vi "IMAQdx LL-Snap.vi"(7 "ImgName":string="untitled", 8 "ErrIn":errorcluster) -> (0 "ErrOut":errorcluster, 3 "ImgOut":T1)   [LabVIEW 2013]
doc: "Use this template to build a VI to use as a subVI."
uses:
  <vilib>/vision/Image Controls.llb/IMAQ Image.ctl
  <vilib>/vision/driver/IMAQdx.llb/IMAQdx Acquisition Mode.ctl
  <vilib>/vision/driver/IMAQdx.llb/IMAQdx Buffer Number Mode.ctl
  <vilib>/vision/driver/NI_Vision_Acquisition_Software.lvlib
panel:
  in  "Camera":refnum<k21> caption="IMAQdx Session"
  # "Input Parameters"
  # "Output Parameters"
  # "VI Description:\nThis VI is created to snap a image from imaging device."
  # ":: MVI Framework V1.0 ::\nAuthor:Gaoke Yang\nEmail: gaoke.yang@yahoo.com\nWeb: www.mvicontrol.com\nCopyright (C) 2013, MVI Technologies All Rights Reserved"
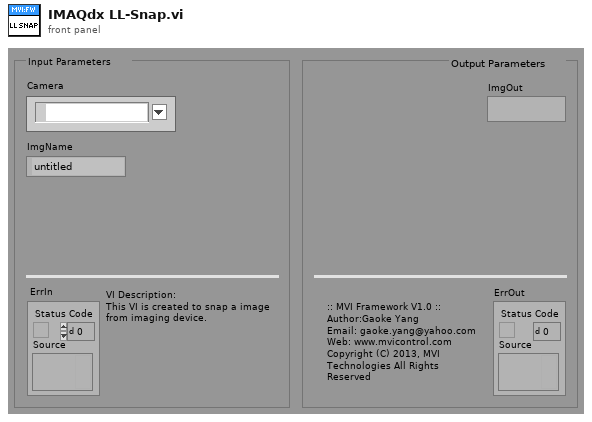
[diagram p1: front panel]
types:
  T1 = typedef "IMAQ Image.ctl" = refnum<image>
  T2 = typedef "NI_Vision_Acquisition_Software.lvlib/IMAQdx Buffer Number Mode.ctl" = enum32{"Next", "Last", "Buffer Number"}
  T3 = typedef "NI_Vision_Acquisition_Software.lvlib/IMAQdx Acquisition Mode.ctl" = enum32{"One Shot", "Continuous"}
  T4 = typedef "IMAQdx.ctl" = refnum<k21>
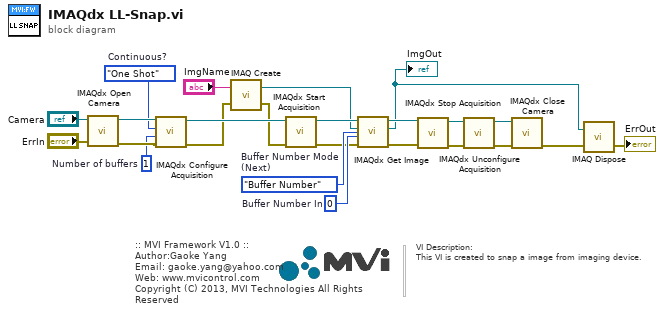
[diagram p0: block diagram]
diagram:
  w8 = u32 0  # Buffer Number In
  w11 = IMAQdx_Buffer_Number_Mode."Buffer Number"  # Buffer Number Mode (Next)
  w17 = IMAQdx_Acquisition_Mode."One Shot"  # Continuous?
  w20 = u32 1  # Number of buffers
  # "VI Description:\nThis VI is created to snap a image from imaging device."
  # ":: MVI Framework V1.0 ::\nAuthor:Gaoke Yang\nEmail: gaoke.yang@yahoo.com\nWeb: www.mvicontrol.com\nCopyright (C) 2013, MVI Technologies All Rights Reserved"
  n1 = call <vilib>:"IMAQdx Open Camera.vi"("error in"="ErrIn", "Session In"="Camera") -> ("error out"=w24:errorcluster, "Session Out"=w18:T4)  [unwired: 8 in]
  n2 = call <vilib>:"IMAQdx Configure Acquisition.vi"("error in"=w24, "Number of Buffers"=w20, "Continuous?"=w17, "Session In"=w18) -> ("error out"=w2:errorcluster, "Session Out"=w12:T4)  [unwired: 6 in]
  n3 = call "IMAQ Create"("Image Name"="ImgName", "error in (no error)"=w2) -> ("New Image"=w3:T1, "error out"=w1:errorcluster)  [unwired: 2 in, 1 out]
  n4 = call <vilib>:"IMAQdx Start Acquisition.vi"("error in"=w1, "Session In"=w12) -> ("error out"=w4:errorcluster, "Session Out"=w5:T4)  [unwired: 8 in]
  n5 = call <vilib>:"IMAQdx Get Image.vi"("Buffer Number Mode (Next)"=w11, "error in"=w4, "Buffer Number In"=w8, "Image In"=w3, "Session In"=w5) -> ("error out"=w10:errorcluster, "Image Out"=w6:T1, "Session Out"=w7:T4)  [unwired: 4 out]
  "ImgOut" <- w6
  n6 = call <vilib>:"IMAQdx Stop Acquisition.vi"("error in"=w10, "Session In"=w7) -> ("error out"=w15:errorcluster, "Session Out"=w16:T4)  [unwired: 8 out]
  n7 = call <vilib>:"IMAQdx Unconfigure Acquisition.vi"("error in"=w15, "Session In"=w16) -> ("error out"=w14:errorcluster, "Session Out"=w13:T4)  [unwired: 8 out]
  n8 = call <vilib>:"IMAQdx Close Camera.vi"("error in"=w14, "Session In"=w13) -> ("error out"=w9:errorcluster)  [unwired: 9 out]
  n9 = call "IMAQ Dispose"("Image"=w6, "error in (no error)"=w9) -> ("error out"=→"ErrOut":errorcluster)  [unwired: 1 in, 3 out]
